vi "USRP Rx Streaming (Host).vi"() -> ()   [LabVIEW 2016]
doc: "This template is for the Simple NI-USRP Streaming design, a design that shows the basics of streaming data to and from an NI USRP-294x/295x device. Refer to the block diagram for more information about how to use this template."
uses:
  <vilib>/userdefined/Silver/nirio_resource_slv.ctl
  Host/SubVIs/USRP Start Trigger.ctl
  Host/SubVIs/USRP Rx Channels.ctl
panel:
  in  "Graph?":bool
  out "Iterations":i32
  out "Number of Warnings":u64
  out "Error Out":errorcluster
  in  "config tab":enum32{"Rx Configuration"}(tab)
  in  "rx config":T2={"rf enable 0"=TRUE, "rf config 0"={"antenna"="RX2", "frequency"=2000000000.0, "lo frequency"=-1.0, "level"=0.0}, "rf enable 1"=TRUE, "rf config 1"={"antenna"="RX2", "frequency"=2000000000.0, "lo frequency"=-1.0, "level"=0.0}, "transfer mode"=enum."Continuous", "sample rate"=10000000.0, "number of samples"=8192, "start trigger"=enum."Immediate"} {"sample rate" format="%#.3pS/s"; "rf config 1"."level" format="%#_gdBm"; "rf config 1"."lo frequency" format="%#.3pHz"; "rf config 1"."frequency" format="%#.3pHz"; "rf config 0"."level" format="%#_gdBm"; "rf config 0"."lo frequency" format="%#.3pHz"; "rf config 0"."frequency" format="%#.3pHz"}
  in  "rx.stop":bool
  out "acquiring":bool caption="Acquiring"
  in  "USRP RIO device":T3="PXI2Slot18Port1Dev1" caption="USRP RIO Device"
  in  "reference frequency source":string(combo)="Internal" caption="Reference Frequency Source"
  in  "indicator tab":T4(tab)
  out "power spectrum":cluster{"f0":dbl, "df":dbl, "magnitude":dbl[]}[](graph) caption="Power Spectrum"
  out "power level":dbl[][](graph) caption="Power Level"
  out "iq data":waveform(dbl)[](graph) caption="I & Q Data"
  out "rx.coerced config":T5 caption="Rx" {"coerced sample rates" format="%#.3pS/s"; "coerced levels" format="%#.3gdBm"; "coerced lo frequencies" format="%#.3pHz"; "coerced frequencies" format="%#.3pHz"}
  # "Simple Rx Streaming"
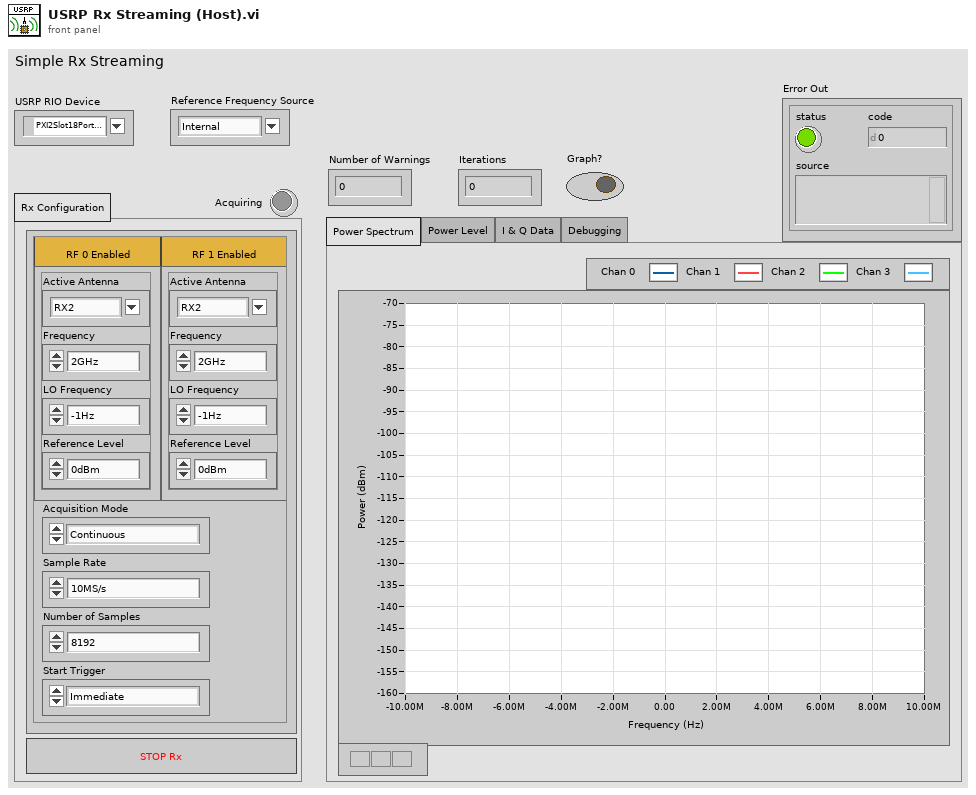
[diagram p1: front panel]
types:
  T1 = typedef "USRP Start Trigger.ctl" = enum8{"Software", "Digital Edge", "Rx Start Trigger", "Tx Start Trigger", "Immediate", "Future Time Event"}
  T2 = cluster{"rf enable 0":bool, "rf config 0":cluster{"antenna":string, "frequency":dbl, "lo frequency":dbl, "level":dbl}, "rf enable 1":bool, "rf config 1":cluster{"antenna":string, "frequency":dbl, "lo frequency":dbl, "level":dbl}, "transfer mode":enum16{"Finite", "Continuous"}, "sample rate":dbl, "number of samples":u32, "start trigger":T1}
  T3 = typedef "nirio_resource_slv.ctl" = tag
  T4 = enum32{"Power Spectrum", "Power Level", "I & Q Data", "Debugging"}
  T5 = cluster{"coerced frequencies":dbl[], "coerced lo frequencies":dbl[], "coerced levels":dbl[], "coerced sample rates":dbl[]}
  T6 = cluster{"daughterboard 0 lo configuration":enum16{"Independent", "Import", "Shared and Export"}, "daughterboard 1 lo configuration":enum16{"Independent", "Import", "Shared and Export"}}
  T7 = typedef "USRP Rx Channels.ctl" = cluster{"rx config":cluster{"channel configuration":cluster{"channel enable":bool, "channel configuration":cluster{"antenna":string, "frequency":dbl, "lo frequency":dbl, "level":dbl}}[], "transfer mode":enum16{"Finite", "Continuous"}, "sample rate":dbl, "number of samples":u32, "start trigger":T1}, "reference frequency source":string, "rx.data sink":enum16{"SFP Port 0", "SFP Port 1", "Host"}, "rx.enabled channels":string[], "vertical range":dbl[], "rx.coerced configurations":cluster{"coerced frequencies":dbl[], "coerced lo frequencies":dbl[], "coerced levels":dbl[], "coerced sample rates":dbl[]}}
  T8 = cluster{"channel configuration":cluster{"channel enable":bool, "channel configuration":cluster{"antenna":string, "frequency":dbl, "lo frequency":dbl, "level":dbl}}[], "transfer mode":enum16{"Finite", "Continuous"}, "sample rate":dbl, "number of samples":u32, "start trigger":T1, "tone frequency":dbl}
  T9 = cluster{"channel configuration":cluster{"channel enable":bool, "channel configuration":cluster{"antenna":string, "frequency":dbl, "lo frequency":dbl, "level":dbl}}[], "transfer mode":enum16{"Finite", "Continuous"}, "sample rate":dbl, "number of samples":u32, "start trigger":T1}
  T10 = typedef "niUsrpRio Config v1 Host.lvlib/niUsrpRio Session.ctl" = cluster{"FPGA Interface":refnum<k20>, "RIO Interface Number":u32, "Data Clock Rate":u32, "FPGA Data Clock Rate":u32, "Global Settings Register Bus":T11, "Radio 0 Settings Register Bus":T11, "Radio 1 Settings Register Bus":T11, "Radio Settings Bus Semaphore":T12, "DB Queues":T13[], "Characterization Data Valid?":bool, "EEPROM Header":T14, "Device Data Header":T15, "EEPROM Characterization Header":T16, "Characterization Data":T17[], "FPGA Current Version":u32, "FPGA Oldest Compatible Version":u32, "Fixed Logic Current Version":u32, "Fixed Logic Oldest Compatible Version":u32, "FPGA Radio Settings Bus Current Version":u32, "FPGA Radio Settings Bus Oldest Compatible Version":u32, "FPGA Board Config Current Version":u32, "FPGA Board Config Oldest Compatible Version":u32, "Daughterboard Clock Rate":u32, "daughterboard configuration session handles":u64[]}
  T11 = typedef "niInstr Register Bus v0 Host.lvlib/Register Bus Session.ctl" = refnum<queue>
  T12 = typedef "Semaphore RefNum" = refnum<k1>
  T13 = typedef "niUsrpRio Config v1 Host.lvlib/DB Queue Reference.ctl" = refnum<queue>
  T14 = typedef "niUsrpRio Config v1 Host.lvlib/EEPROM Header.ctl" = cluster{"Checksum":u32, "Product Code":u16, "Hardware Current Version":u16, "Hardware Oldest Compatible Version":u16, "EEPROM Map Current Version":u16, "EEPROM Map Oldest Compatible Version":u16, "User Password":string, "Pointer to Factory Header":u32, "Pointer to User Header":u32, "Recommended Interval":u16, "Number of Reserved Bytes":i32, "Number of Daughterboards":u8, "Daughterboard IDs":u16[], "Daughterboard Serial Numbers":string[]}
  T15 = typedef "niUsrpRio Config v1 Host.lvlib/EEPROM Device Data Header.ctl" = cluster{"Checksum":u32, "Number of Channels":u8, "Number of Gain Settings":u16[], "Pointer to Characterization Data":u32[], "Number of Reserved Bytes":i32, "Number of Frequencies":u16[]}
  T16 = typedef "niUsrpRio Config v1 Host.lvlib/EEPROM Characterization Header.ctl" = cluster{"Checksum":u32, "Date":timestamp, "Temperature":sgl, "Misc. Info":string, "Pointer to Device Data Header":u32, "Number of Reserved Bytes":i32}
  T17 = typedef "niUsrpRio Config v1 Host.lvlib/Characterization Data.ctl" = cluster{"Gains[dB]":dbl[], "Frequencies [Hz]":dbl[], "IQ Imbalance Table":T18[], "Measured Gains[dB]":dbl[][]}
  T18 = typedef "niUsrpRio Config v1 Host.lvlib/IQ Imbalance.ctl" = cluster{"Gain Imbalance [linear]":dbl, "Phase Imbalance [radians]":dbl, "Offset":cdb}
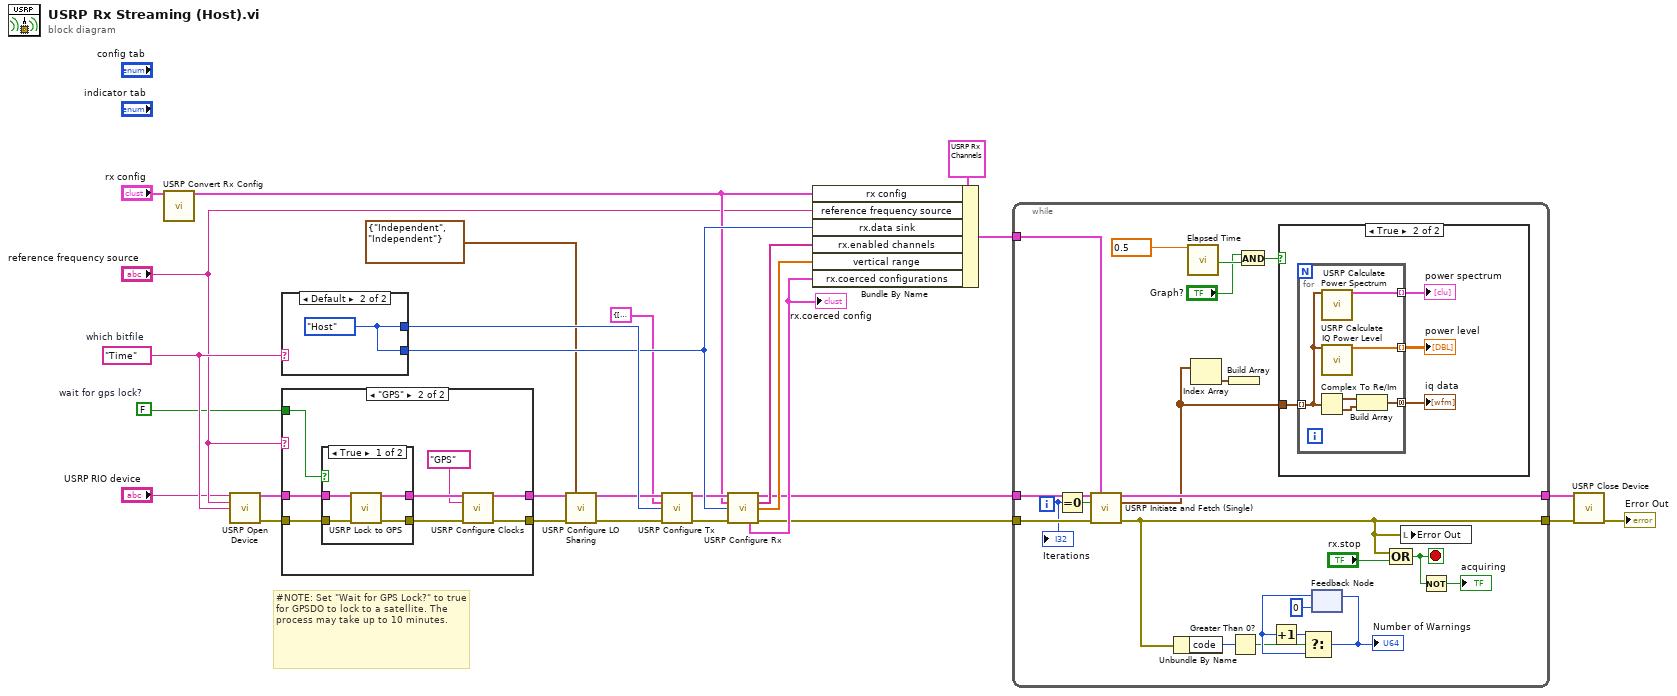
[diagram p0: block diagram]
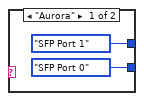
[diagram p2: hidden frame]
diagram:
  w6 = FALSE  # wait for gps lock?
  w8 = "Time"  # which bitfile
  # "#NOTE: Set \"Wait for GPS Lock?\" to true for GPSDO to lock to a satellite. The process may take up to 10 minutes."
  n1 = call "USRP Convert Rx Config.vi"("rx config"="rx config") -> ("rx config out"=w10:T9)  [unwired: 14 in]
  n2 = call "USRP Open Device.vi"("USRP RIO device"="USRP RIO device", "Reference Frequency Source"="reference frequency source", "which bitfile"=w8) -> ("niUsrpRio Session (out)"=w17:T10, "error out"=w16:errorcluster)  [unwired: 11 in]
  n3 = case shown="Default" w8 {
    tunnel: [enum16{"SFP Port 0", "SFP Port 1", "Host"}."SFP Port 1" ("data stream config") w31] -> w23
    tunnel: [enum16{"SFP Port 0", "SFP Port 1", "Host"}."SFP Port 0" ("data stream config") w31] -> w22
    frame "Aurora" {
    }
    frame Default {
      w31 = enum16{"SFP Port 0", "SFP Port 1", "Host"}."Host" ("data stream config")
    }
  }
  n4 = case shown="\"GPS\"" "reference frequency source" {
    tunnel: w17 -> [w33 w41]
    tunnel: [w33 w36] -> w14
    tunnel: [w32 w38] -> w13
    tunnel: w16 -> [w32 w40]
    tunnel: w6 -> [_ w34]
    frame Default {
    }
    frame "GPS" {
      n5 = case shown="True" w34 {
        tunnel: w41 -> [w43 w47]
        tunnel: [w45 w47] -> w37
        tunnel: [w44 w46] -> w39
        tunnel: w40 -> [w42 w46]
        frame True {
          n6 = call "USRP Lock to GPS.vi"("niUsrpRio Session"=w43, "error in"=w42) -> ("niUsrpRio Session (out)"=w45:T10, "error out"=w44:errorcluster)  [unwired: 12 in]
        }
        frame False {
        }
      }
      n7 = call "USRP Configure Clocks.vi"("niUsrpRio Session"=w37, "Reference Frequency Source"="GPS", "error in"=w39) -> ("niUsrpRio Session (out)"=w36:T10, "error out"=w38:errorcluster)  [unwired: 11 in]
    }
  }
  n8 = call "USRP Configure LO Sharing.vi"("niUsrpRio Session in"=w14, "lo config"=T6 {"daughterboard 0 lo configuration"=enum."Independent", "daughterboard 1 lo configuration"=enum."Independent"}, "error in"=w13) -> ("niUsrpRio Session out"=w15:T10, "error out"=w12:errorcluster)  [unwired: 11 in]
  n9 = call "USRP Configure Tx.vi"("niUsrpRio Session"=w15, "tx config"=T8 {"channel configuration"=[], "transfer mode"=enum."Finite", "sample rate"=10000000.0, "number of samples"=8192, "start trigger"=enum."Immediate", "tone frequency"=100000.0}, "tx.data source"=w23, "error in"=w12) -> ("niUsrpRio Session (out)"=w18:T10, "error out"=w19:errorcluster)  [unwired: 5 in, 5 out]
  n10 = call "USRP Configure Rx.vi"("niUsrpRio Session"=w18, "rx config"=w10, "rx.data sink"=w22, "error in"=w19) -> ("niUsrpRio Session (out)"=w3:T10, "rx.enabled channels"=w21:string[], "vertical range"=w20:dbl[], "rx.coerced configurations"=w4:T5, "error out"=w2:errorcluster)  [unwired: 7 in]
  "rx.coerced config" <- w4
  n11 = Bundle By Name(cluster=T7 {"rx config"={"channel configuration"=[], "transfer mode"=enum."Finite", "sample rate"=10000000.0, "number of samples"=8192, "start trigger"=enum."Immediate"}, "reference frequency source"="Internal", "rx.data sink"=enum."Host", "rx.enabled channels"=[], "vertical range"=[], "rx.coerced configurations"={"coerced frequencies"=[], "coerced lo frequencies"=[], "coerced levels"=[], "coerced sample rates"=[]}} ("rx channels"), "rx config"=w10, "reference frequency source"="reference frequency source", "rx.data sink"=w22, "rx.enabled channels"=w21, "vertical range"=w20, "rx.coerced configurations"=w4) -> (w1:T7)
  n12 = while {
    tunnel: w3 -> [w67]
    tunnel: [w66] -> w27
    tunnel: w1 -> [w63]
    tunnel: w2 -> [w68]
    tunnel: [w55] -> w28
    i -> [w52]
    stop <- w64 stop-if-true
    # "Acquire and Fetch a waveform"
    n13 = Equal To 0?(x=w52) -> (x = 0?=w60:bool)
    n14 = call "USRP Initiate and Fetch (Single).vi"("niUsrpRio Session"=w67, "rx channels"=w63, "first iteration"=w60, "error in"=w68) -> ("niUsrpRio Session (out)"=w66:T10, "complex baseband data"=w48:waveform(cdb)[], "error out"=w55:errorcluster)  [unwired: 9 in]
    n15 = Unbundle By Name(w55) -> ("code"=w54:i32)
    n16 = call "Elapsed Time"("Time Target (s)"=0.5 ("retrigger delay")) -> ("Time has Elapsed"=w62:bool)  [unwired: 11 in, 7 out]
    n17 = Index Array(array=w48) -> (element=w51:waveform(cdb))  [unwired: 1 in]
    n18 = Build Array(w51) -> ()  [unwired: 1 out]
    n19 = Greater Than 0?(x=w54) -> (x > 0?=w53:bool)
    n20 = And(x="Graph?", y=w62) -> (x .and. y?=w50:bool)
    n21 = case shown="True" w50 {
      tunnel: w48 -> [_ w73]
      frame False {
      }
      frame True {
        n22 = for {
          tunnel: [w77] -> w72 mode=concatenating
          tunnel: [w76] -> w71 mode=indexing
          tunnel: [w75] -> w70 mode=indexing
          tunnel: w73 -> [w74] mode=indexing
          n23 = Complex To Re/Im(x + iy=w74) -> (x=w79:waveform(dbl), y=w78:waveform(dbl))
          n24 = call "USRP Calculate Power Spectrum.vi"("waveform"=w74) -> ("power spectrum (dBm)"=w75:cluster{"f0":dbl, "df":dbl, "magnitude":dbl[]})  [unwired: 14 in]
          n25 = call "USRP Calculate IQ Power Level.vi"("iq data"=w74) -> ("power level (dBm)"=w76:dbl[])  [unwired: 14 in]
          n26 = Build Array(w79, w78) -> (w77:waveform(dbl)[])
        }
        "power level" <- w71
        "power spectrum" <- w70
        "iq data" <- w72
      }
    }
    n27 = feedback #1(u64 0) -> (w59:u64)
    n28 = Increment(x=w59) -> (x+1=w58:u64)
    n29 = Select(t=w58, s=w53, f=w59) -> (s? t:f=w56:u64)
    "Number of Warnings" <- w56
    n30 = feedback-in #1(w56) -> ()
    n31 = Compound Arithmetic op=OR(w55, "rx.stop") -> (w64:bool)
    n32 = local write "Error Out"(w55) -> ()
    n33 = Not(x=w64) -> (.not. x?=→"acquiring":bool)
    "Iterations" <- w52
  }
  n34 = call "USRP Close Device.vi"("niUsrpRio Session"=w27, "error in"=w28) -> ("error out"=→"Error Out":errorcluster)  [unwired: 13 in]
